vi "RestartSensor.vi"(8 "error in (no error)":errorcluster, 9 "milliseconds to wait":u32=2000, 10 "Address":u8, 11 "VISA resource name":refnum<visa-resource-name>) -> (0 "error out":errorcluster, 3 "VISA resource name out":refnum<visa-resource-name>)   [LabVIEW 2020, in "driver_flodx_ph_probe.lvlib"]
doc: "Restarts the pH probe, after restarting you will need to reintialize communications."
uses:
  <instrlib>/RxnRover/FloDx Ph Probe Driver/driver_flodx_ph_probe.lvlib
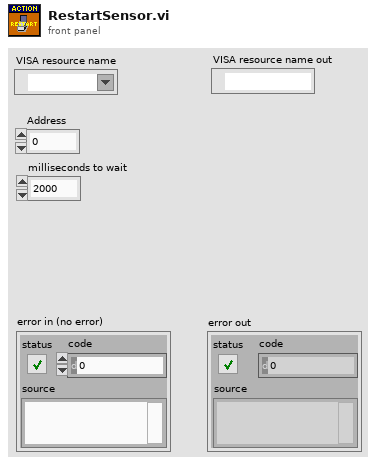
[diagram p1: front panel]
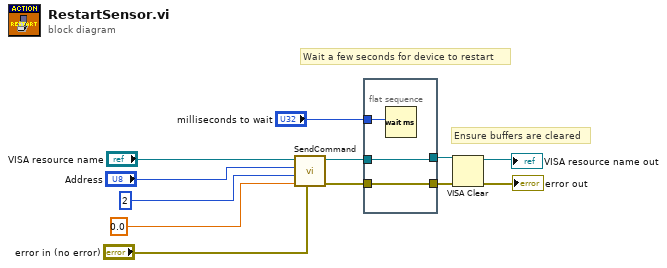
[diagram p0: block diagram]
diagram:
  # "Ensure buffers are cleared"
  # "Wait a few seconds for device to restart"
  n1 = call <instrlib>:"SendCommand.vi"("error in"="error in (no error)", "Parameter"=sgl 0.0, "Command"=u8 2, "Address"="Address", "VISA resource name"="VISA resource name") -> ("error out"=w7:errorcluster, "VISA resource name out"=w6:refnum<visa-resource-name>)  [unwired: 4 in, 1 out]
  n2 = flat-sequence {
    tunnel: [w15] -> w1
    tunnel: w7 -> [w15]
    tunnel: [w14] -> w4
    tunnel: w6 -> [w14]
    tunnel: "milliseconds to wait" -> [w13]
    frame #0 {
      n3 = Wait (ms)(milliseconds to wait=w13) -> ()  [unwired: 1 out]
    }
  }
  n4 = VISA Clear(VISA resource name=w4, error in (no error)=w1) -> (VISA resource name out=→"VISA resource name out":refnum<visa-resource-name>, error out=→"error out":errorcluster)
